vi "EEPROM读写实验.vi"() -> ()   [LabVIEW 2011]
uses:
  <vilib>/STM32_DriverVI_Interface_F4/IIC/IIC_Select_F4.ctl
  <vilib>/STM32_DriverVI_Interface_F4/LCD/Show_Mode_F4.ctl
  <vilib>/STM32_DriverVI_Interface_F4/LCD/Font_Size_F4.ctl
  <vilib>/STM32_DriverVI_Interface_F4/LCD/Brush Color_Index_F4.ctl
  <vilib>/eio/EIO_TerminalDirection.ctl
  <vilib>/STM32_DriverVI_Interface_F4/LCD/LCD_Init_F4.vi
  <vilib>/STM32_DriverVI_Interface_F4/GPIO_EIO/GPI_EIO_Inner_F4.vi
  <vilib>/eio/EIONode/EIONode.xnode
panel:
  in  "Number Byte":u16
  out "字符串":string
  in  "x":bool
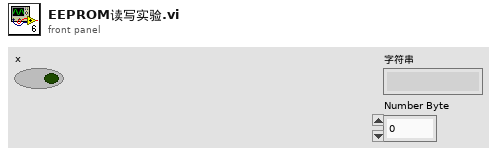
[diagram p1: front panel]
types:
  T1 = enum8{"P0", "P1", "P2", "P3", "P4", "P5", "P6", "P7", "P8", "P9", "P10", "P11", "P12", "P13", "P14", "P15"}
  T2 = enum8{"Port_A", "Port_B", "Port_C", "Port_D", "Port_E", "Port_F", "Port_G", "Port_H", "Port_I"}
  T3 = typedef "IIC_Select_F4.ctl" = enum8{"IIC_Group_1", "IIC_Group_2", "IIC_Group_3", "IIC_Group_4", "IIC_Group_5", "IIC_Group_6", "IIC_Group_7", "IIC_Group_8"}
  T4 = typedef "Show_Mode_F4.ctl" = enum8{"非叠加显示", "叠加显示"}
  T5 = typedef "Font_Size_F4.ctl" = enum8{"Small_Font（12）", "Big_Font（16）"}
  T6 = typedef "Brush Color_Index_F4.ctl" = enum8{"White", "Black", "Blue", "Green_Blue", "Red", "Magenta（品红）", "Green", "Cyan（青色）", "Yellow", "Brown", "Brown_Red", "Gray", "Dark_Blue", "Light_Blue", "Gray_Blue", "Light_Green", "Light_Gray", "Light_Gray_Blue", "Light_Brown_Blue"}
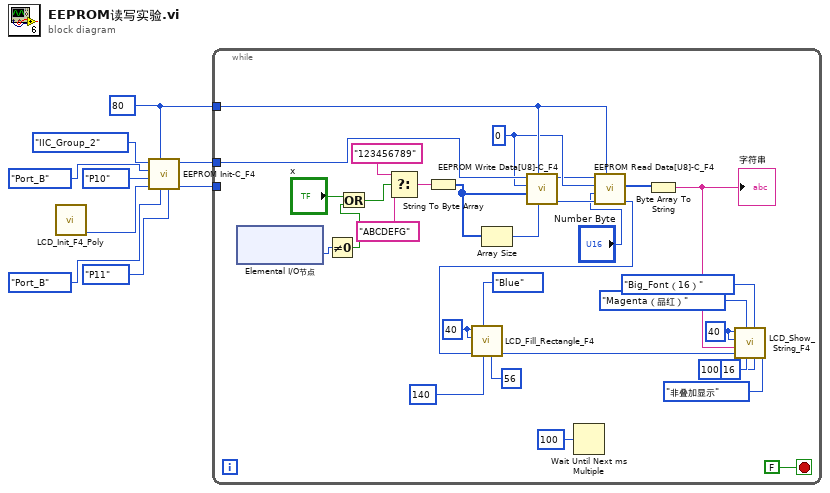
[diagram p0: block diagram]
diagram:
  w1 = u8 80 ("器件地址（7位）")
  n1 = call-poly <vilib>:"LCD_Init_F4_Poly.vi"() -> ("err_out"=w2:u8)  [unwired: 10 in, 1 out]
  n2 = call <vilib>:"EEPROM Init-C_F4.vi"("SDA_pin"=T1."P11", "SDA_PortX"=T2."Port_B", "器件地址（7位）"=w1, "err_in"=w2, "SCL_pin"=T1."P10", "SCL_PortX"=T2."Port_B", "IIC_Select"=IIC_Select_F4."IIC_Group_2") -> ("err_out"=w7:u8, "IIC_Reference_Out"=w6:u16)  [unwired: 2 in, 1 out]
  n3 = while {
    tunnel: w6 -> [w30]
    tunnel: w7 -> [_]
    tunnel: w1 -> [w32]
    stop <- FALSE stop-if-true
    w18 = u16 40 ("X_Position")
    w22 = u16 40 ("X1_Position")
    w29 = u16 0 ("Address")
    n4 = xnode "Elemental I/O节点"() -> ("KEY_UP"=w12:u8)  [unwired: 1 in, 1 out]
    n5 = Not Equal To 0?(x=w12) -> (x != 0?=w40:bool)
    n6 = Or(x="x", y=w40) -> (x .or. y?=w38:bool)
    n7 = Select(t="123456789", s=w38, f="ABCDEFG") -> (s? t:f=w35:string)
    n8 = String To Byte Array(string=w35) -> (unsigned byte array=w31:u8[])
    n9 = Array Size(array=w31) -> (size(s)=w34:i32)
    n10 = call <vilib>:"EEPROM Write Data[U8]-C_F4.vi"("Length"=w34, "器件地址（7位）"=w32, "Write Data[U8]"=w31, "Address"=w29, "IIC_Reference_In"=w30) -> ("err_out"=w33:u8, "IIC_Reference_Out"=w10:u16)  [unwired: 5 in]
    n11 = Wait Until Next ms Multiple(millisecond multiple=u32 100 ("毫秒倍数")) -> ()  [unwired: 1 out]
    n12 = call <vilib>:"EEPROM Read Data[U8]-C_F4.vi"("器件地址（7位）"=w32, "err_in"=w33, "Number Byte"="Number Byte", "Address"=w29, "IIC_Reference_In"=w10) -> ("err_out"=w26:u8, "Read Data[U8]"=w28:u8[])  [unwired: 4 in, 1 out]
    n13 = call <vilib>:"LCD_Fill_Rectangle_F4.vi"("Y2_Position"=u16 56, "X2_Position"=u16 140, "Brush Color"=Brush_Color_Index_F4."Blue", "err_in"=w26, "Y1_Position"=w22, "X1_Position"=w22) -> ("err_out"=w25:u8)  [unwired: 5 in]
    n14 = Byte Array To String(unsigned byte array=w28) -> (string=w27:string)
    "字符串" <- w27
    n15 = call <vilib>:"LCD_Show_String_F4.vi"("Show_Mode"=Show_Mode_F4."非叠加显示", "Height"=u16 16, "Font_Size"=Font_Size_F4."Big_Font（16）", "Width"=u16 100, "Brush Color"=Brush_Color_Index_F4."Magenta（品红）", "err_in"=w25, "String"=w27, "Y_Position"=w18, "X_Position"=w18) -> ()  [unwired: 2 in, 1 out]
  }
